vi "Autonomous Independent.vi"() -> ()   [LabVIEW 2014]
doc: "This VI is called when autonomous begins, and will automatically be terminated when autonomous ends. You can carry out timed or sensor driven robot movement independently without needing to return to the caller."
uses:
  <vilib>/Rock Robotics/WPI/Joystick/WPI_JoystickGetSetRefNum.vi
  <vilib>/Rock Robotics/Network Tables/SD Write Numeric Array.vi
  <vilib>/Rock Robotics/WPI/RobotDrive/WPI_RobotDriveGetSetRefNum.vi
  <vilib>/Rock Robotics/WPI/RobotDrive/WPI_RobotDriveMecanumDrive_Cartesian.vi
panel:
  out "Right Rear":dbl
  out "Left Rear":dbl
  out "Right Front":dbl
  out "left Front":dbl
  in  "Deceleration Rate":dbl
  in  "Stop Point":dbl
  in  "Default Output":dbl
  out "Y output":dbl(graph)
  out "Y output":dbl
  in  "Reset Encoder":bool
  in  "Reset Gyro":bool
  out "Angle":dbl
  in  "Angle Constant":dbl
  in  "Angular Rate?":bool
  out "left rear":dbl
  out "left front":dbl
  out "right rear":dbl
  out "right front":dbl
  out "Angular Rate":dbl
  out "average":dbl
  out "Left Rear Encoder 3":dbl
  out "Left Front Encoder 3":dbl
  out "Right Rear Encoder 3":dbl
  out "Right Front Encoder 3":dbl
  out "Average 3":dbl
  out "Gyro 3":dbl
  out "Left Rear Encoder 2":dbl
  out "Left Front Encoder 2":dbl
  out "Right Rear Encoder 2":dbl
  out "Right Front Encoder 2":dbl
  out "Average 2":dbl
  out "Gyro 2":dbl
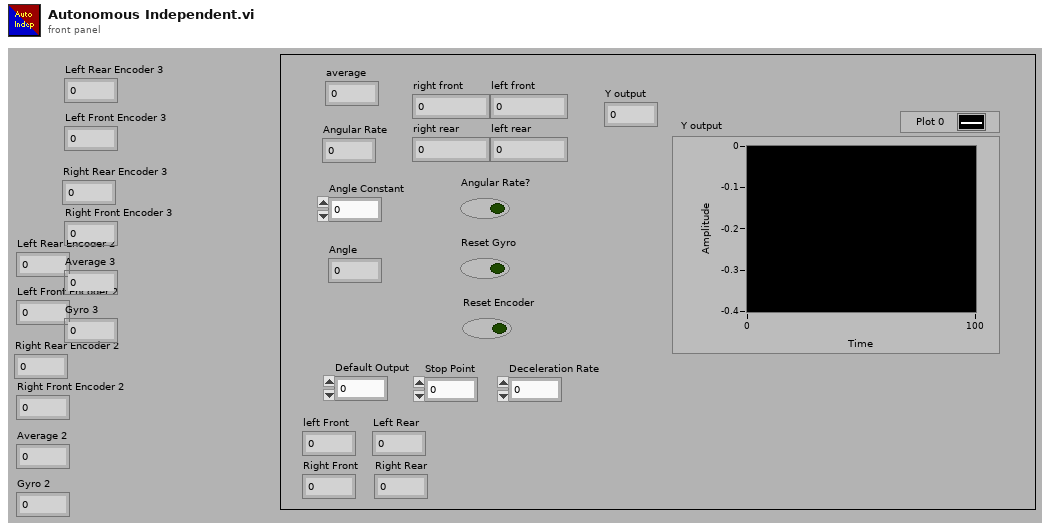
[diagram p1: front panel]
types:
  T1 = typedef "WPI_EncoderDevRef.ctl" = cluster{"DevStatus":errorcluster, "EncoderIndex":T2, "CounterIndex":T3, "DistancePerCount":dbl, "Decoding Type":T4}
  T2 = typedef "FPGA_EncoderIdx.ctl" = enum8{"Enc 0", "Enc 1", "Enc 2", "Enc 3", "Enc 4", "Enc 5", "Enc 6", "Enc 7", "Invalid"}
  T3 = typedef "FPGA_CounterCtrSystemIndex.ctl" = enum8{"Ctr 0", "Ctr 1", "Ctr 2", "Ctr 3", "Ctr 4", "Ctr 5", "Ctr 6", "Ctr 7", "Invalid"}
  T4 = typedef "WPI_EncoderType.ctl" = enum16{"1x", "2x", "4x"}
  T5 = typedef "WPI_GyroDevRef.ctl" = cluster{"DevStatus":errorcluster, "Analog Module":T6, "Analog Channel":T7, "Offset":dbl, "Gain (VoltsPerDegree/Second)":dbl}
  T6 = typedef "FPGA_TypedefAnalogModule.ctl" = enum16{"Controller 1"}
  T7 = typedef "FPGA_AIChannel.ctl" = enum8{"AI 0", "AI 1", "AI 2", "AI 3", "AI MXP 0", "AI MXP 1", "AI MXP 2", "AI MXP 3", "Invalid"}
  T8 = typedef "WPI_RobotDriveDevRef.ctl" = cluster{"DevStatus":errorcluster, "Motors[]":T9[], "Square Inputs":bool, "Max Output":dbl}
  T9 = typedef "WPI_MotorControlDeviceRef.ctl" = cluster{"DeviceStatus":errorcluster, "Type":T10, "PWM":cluster{"Controller":T11, "PWM Channel":T12, "DeadBand":T13}, "CAN":cluster{"Device Number":u8, "Control Mode":T14, "Semaphore":T15, "Max Vout":dbl, "TalonSRX Control Mode":T16}, "Invert":bool, "TransformRef":T17, "InvTransformRef":T17}
  T10 = typedef "WPI_MotorControlType.ctl" = enum16{"PWM", "CAN", "CANTalonSRX"}
  T11 = typedef "FPGA_TypedefDigitalModule.ctl" = enum16{"Controller 1"}
  T12 = typedef "FPGA_DIOPWMChannel.ctl" = enum8{"PWM 0", "PWM 1", "PWM 2", "PWM 3", "PWM 4", "PWM 5", "PWM 6", "PWM 7", "PWM 8", "PWM 9", "PWM MXP 0", "PWM MXP 1", "PWM MXP 2", "PWM MXP 3", "PWM MXP 4", "PWM MXP 5", "PWM MXP 6", "PWM MXP 7", "PWM MXP 8", "PWM MXP 9", "Invalid"}
  T13 = typedef "WPI_PWMDeadband.ctl" = cluster{"Name":string, "maxPositivePwm":i32, "minPositivePwm":i32, "centerPwm":i32, "maxNegativePwm":i32, "minNegativePwm":i32, "angularRange":u16}
  T14 = typedef "WPI_CANJaguar_ControlMode.ctl" = enum8{"Percent VBus", "Current", "Speed", "Position", "Voltage"}
  T15 = typedef "Semaphore RefNum" = refnum<k1>
  T16 = typedef "WPI_CANTalonSRX_APIControlMode.ctl" = enum8{"Percent VBus", "Speed", "Position", "Slave", "Unchanged / Invalid"}
  T17 = typedef "WPI_PWMTransform_ConPane.ctl" = refnum<vi>
  T18 = typedef "WPI_JoystickDevRef.ctl" = cluster{"Device":T19}
  T19 = typedef "WPI_JoystickDeviceEnum.ctl" = enum16{"USB 0", "USB 1", "USB 2", "USB 3", "USB 4", "USB 5"}
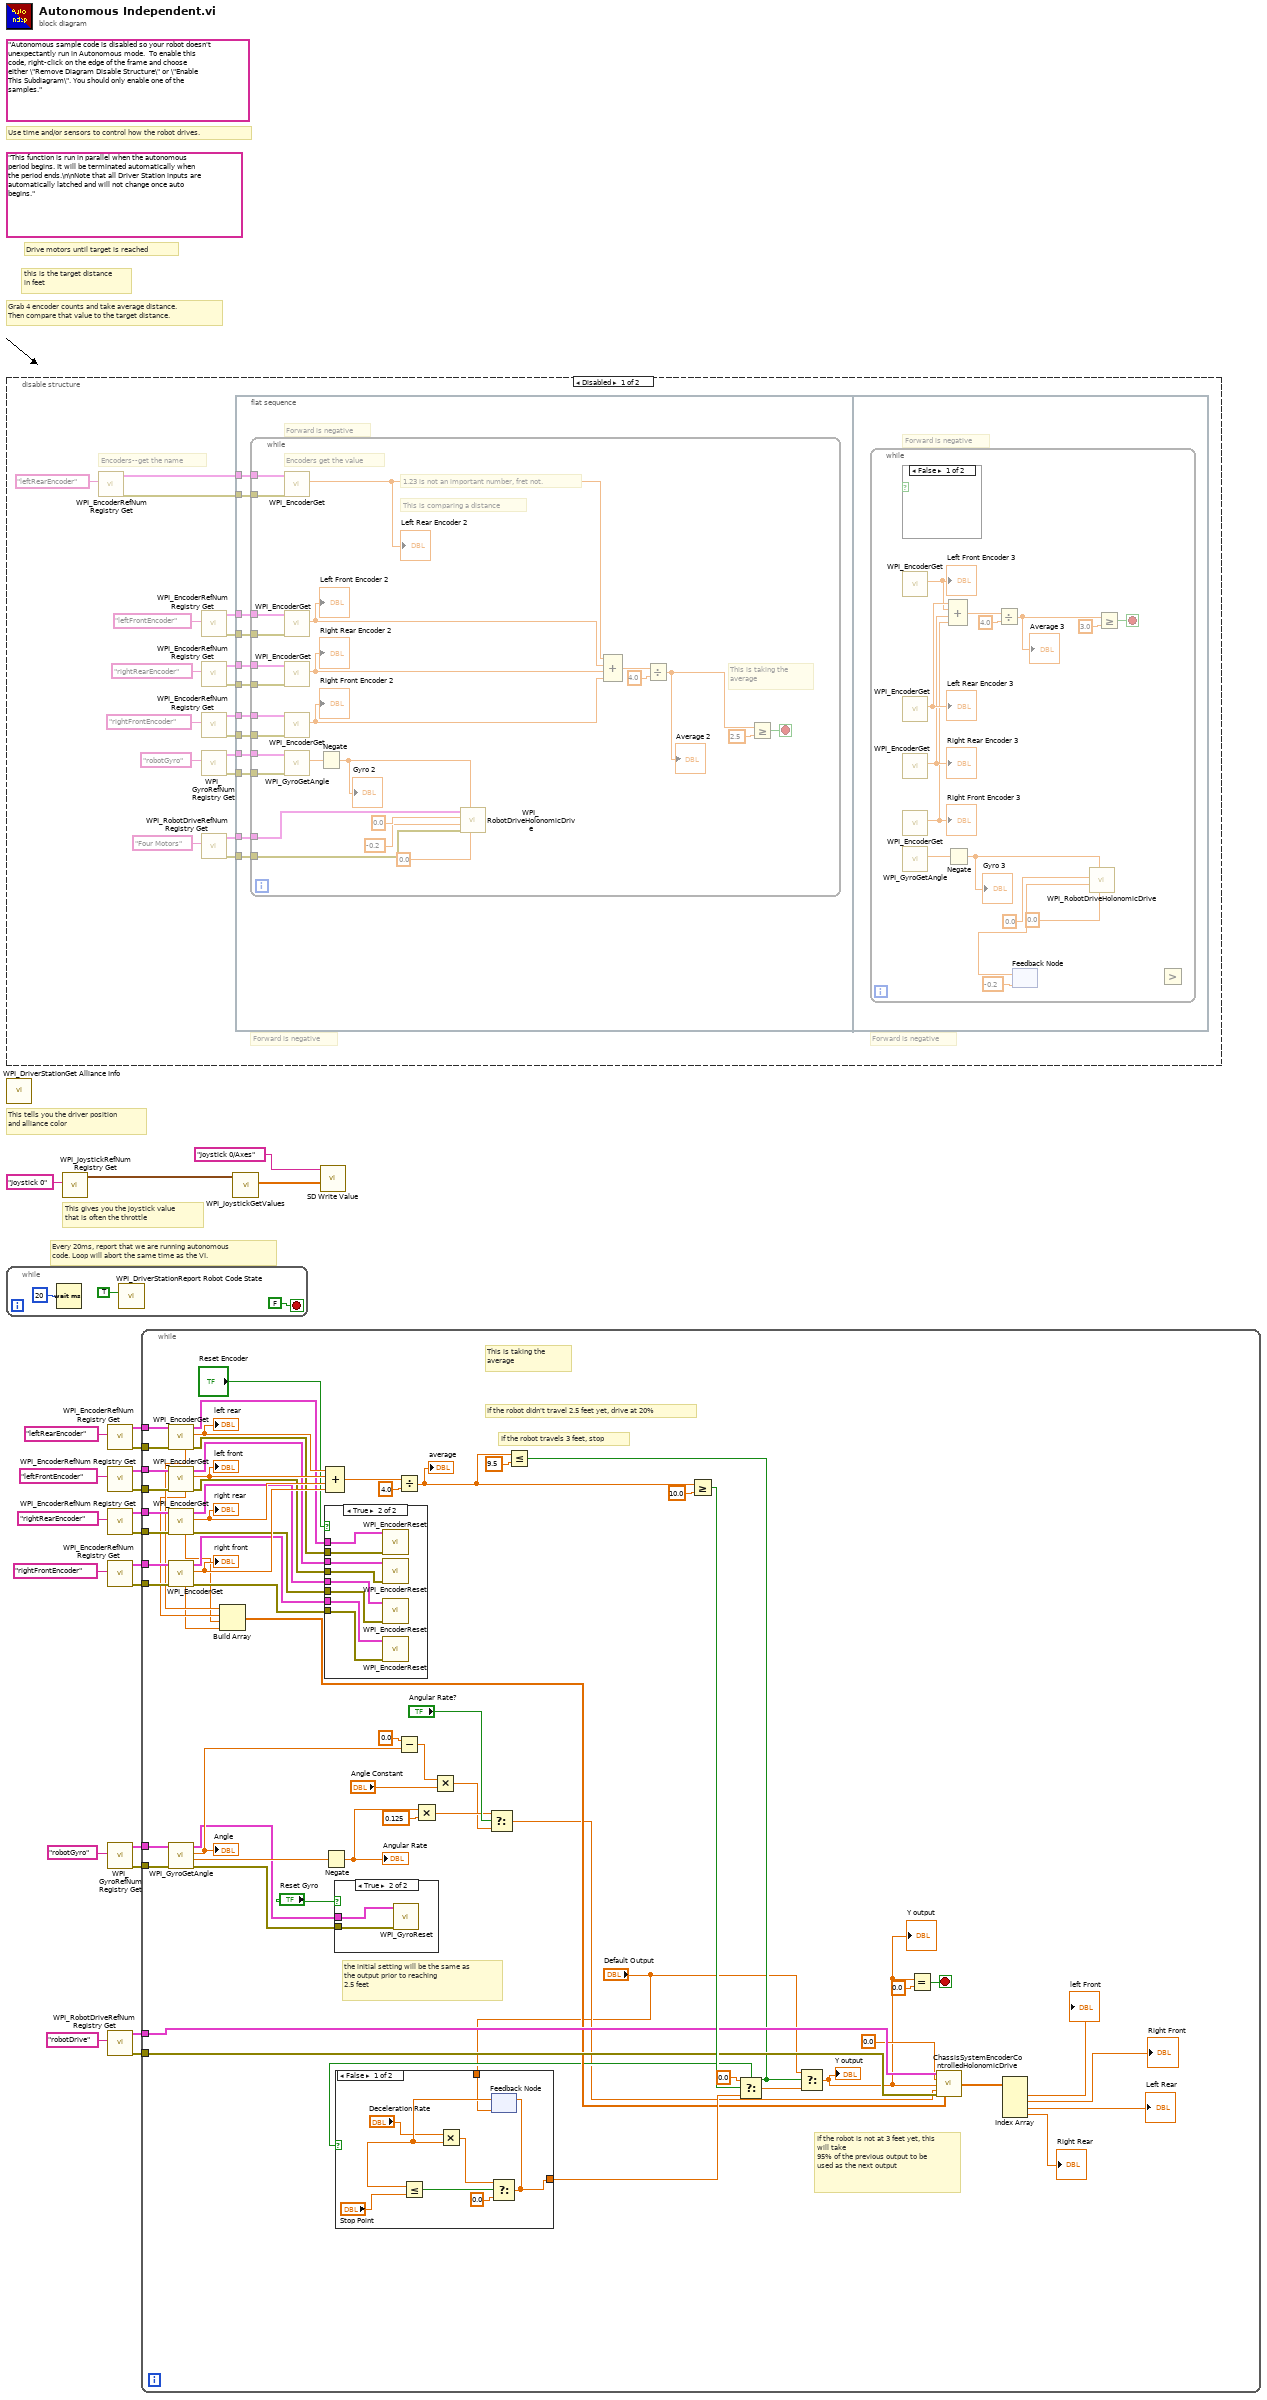
[diagram p0: block diagram]
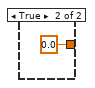
[diagram p2: hidden frame]
diagram:
  (unwired) "Autonomous sample code is disabled so your robot doesn't unexpectantly run in Autonomous mode.  To enable this code, right-click on the edge of the frame and choose either \"Remove Diagram Disable Structure\" or \"Enable This Subdiagram\". You should only enable one of the samples."
  (unwired) "This function is run in parallel when the autonomous period begins. It will be terminated automatically when the period ends.\n\nNote that all Driver Station inputs are automatically latched and will not change once auto begins."
  # "this is the target distance\nin feet"
  # "Drive motors until target is reached"
  # "Grab 4 encoder counts and take average distance.\nThen compare that value to the target distance."
  # "Every 20ms, report that we are running autonomous\ncode. Loop will abort the same time as the VI."
  # "This gives you the joystick value\nthat is often the throttle"
  # "Use time and/or sensors to control how the robot drives."
  # "This tells you the driver position\nand alliance color"
  n1 = disable-structure shown="Disabled" {
    frame Disabled {
      # "Forward is negative"
      # "Forward is negative"
      # "Encoders--get the name"
      n2 = call <vilib>:"WPI_EncoderRefNum Registry Get.vi"("refnum name"="leftRearEncoder") -> ("error out"=w29:errorcluster, "EncoderDevRef"=w30:T1)  [unwired: 9 in]
      n3 = call <vilib>:"WPI_EncoderRefNum Registry Get.vi"("refnum name"="leftFrontEncoder") -> ("error out"=w27:errorcluster, "EncoderDevRef"=w28:T1)  [unwired: 9 in]
      n4 = call <vilib>:"WPI_EncoderRefNum Registry Get.vi"("refnum name"="rightRearEncoder") -> ("error out"=w25:errorcluster, "EncoderDevRef"=w26:T1)  [unwired: 9 in]
      n5 = call <vilib>:"WPI_EncoderRefNum Registry Get.vi"("refnum name"="rightFrontEncoder") -> ("error out"=w24:errorcluster, "EncoderDevRef"=w23:T1)  [unwired: 9 in]
      n6 = call <vilib>:"WPI_GyroRefNum Registry Get.vi"("refnum name"="robotGyro") -> ("error out"=w33:errorcluster, "GyroDevRef"=w34:T5)  [unwired: 9 in]
      n7 = call <vilib>:"WPI_RobotDriveRefNum Registry Get.vi"("refnum name"="Four Motors") -> ("error out"=w31:errorcluster, "RobotDriveDevRef"=w32:T8)  [unwired: 9 in]
      n8 = flat-sequence {
        tunnel: w34 -> [w52]
        tunnel: w33 -> [w51]
        tunnel: w32 -> [w50]
        tunnel: w31 -> [w49]
        tunnel: w30 -> [w48]
        tunnel: w29 -> [w47]
        tunnel: w28 -> [w46]
        tunnel: w27 -> [w45]
        tunnel: w26 -> [w44]
        tunnel: w25 -> [w43]
        tunnel: w24 -> [w42]
        tunnel: w23 -> [w41]
        frame #0 {
          # "Forward is negative"
          n9 = while {
            tunnel: w52 -> [w60]
            tunnel: w51 -> [w59]
            tunnel: w50 -> [w58]
            tunnel: w49 -> [w57]
            tunnel: w48 -> [w71]
            tunnel: w47 -> [w70]
            tunnel: w46 -> [w69]
            tunnel: w45 -> [w68]
            tunnel: w44 -> [w67]
            tunnel: w43 -> [w66]
            tunnel: w41 -> [w65]
            tunnel: w42 -> [w64]
            stop <- w63 stop-if-true
            # "Encoders get the value"
            # "This is comparing a distance"
            # "This is taking the average"
            # "1.23 is not an important number, fret not."
            n10 = call <vilib>:"WPI_EncoderGet.vi"("error in (no error)"=w70, "EncoderDevRef"=w71) -> ("Distance"=w75:dbl)  [unwired: 4 in, 5 out]
            "Left Rear Encoder 2" <- w75
            n11 = call <vilib>:"WPI_EncoderGet.vi"("error in (no error)"=w68, "EncoderDevRef"=w69) -> ("Distance"=w74:dbl)  [unwired: 4 in, 5 out]
            "Left Front Encoder 2" <- w74
            n12 = call <vilib>:"WPI_EncoderGet.vi"("error in (no error)"=w66, "EncoderDevRef"=w67) -> ("Distance"=w73:dbl)  [unwired: 4 in, 5 out]
            "Right Rear Encoder 2" <- w73
            n13 = call <vilib>:"WPI_EncoderGet.vi"("error in (no error)"=w64, "EncoderDevRef"=w65) -> ("Distance"=w72:dbl)  [unwired: 4 in, 5 out]
            "Right Front Encoder 2" <- w72
            n14 = call <vilib>:"WPI_GyroGetAngle.vi"("error in (no error)"=w59, "GyroDevRef"=w60) -> ("Angle"=w56:dbl)  [unwired: 6 in, 3 out]
            n15 = Negate(x=w56) -> (-x=w55:dbl)
            "Gyro 2" <- w55
            n16 = call-poly <vilib>:"WPI_RobotDriveHolonomicDrive.vi"("Rotation"=0.0, "Gyro Angle"=w55, "error in (no error)"=w57, "Y"=-0.2, "X"=0.0, "RobotDriveDevRef"=w58) -> ()  [unwired: 3 in, 3 out]
            n17 = Compound Arithmetic op=ADD(w75, w74, w73, w72) -> (w77:dbl)
            n18 = Divide(x=w77, y=4.0) -> (x/y=w54:dbl)
            "Average 2" <- w54
            n19 = Greater Or Equal?(x=w54, y=2.5) -> (x >= y?=w63:bool)
          }
        }
        frame #1 {
          # "Forward is negative"
          n20 = while {
            stop <- w86 stop-if-true
            n21 = case shown="False" {
              selector: _ -> [_ _]
              frame False {
              }
              frame True {
              }
            }
            n22 = call <vilib>:"WPI_EncoderGet.vi"() -> ("Distance"=w89:dbl)  [unwired: 6 in, 5 out]
            "Left Front Encoder 3" <- w89
            n23 = call <vilib>:"WPI_EncoderGet.vi"() -> ("Distance"=w90:dbl)  [unwired: 6 in, 5 out]
            "Left Rear Encoder 3" <- w90
            n24 = call <vilib>:"WPI_EncoderGet.vi"() -> ("Distance"=w88:dbl)  [unwired: 6 in, 5 out]
            "Right Rear Encoder 3" <- w88
            n25 = call <vilib>:"WPI_EncoderGet.vi"() -> ("Distance"=w87:dbl)  [unwired: 6 in, 5 out]
            "Right Front Encoder 3" <- w87
            n26 = call <vilib>:"WPI_GyroGetAngle.vi"() -> ("Angle"=w83:dbl)  [unwired: 8 in, 3 out]
            n27 = Negate(x=w83) -> (-x=w82:dbl)
            "Gyro 3" <- w82
            n28 = Compound Arithmetic op=ADD(w90, w89, w88, w87) -> (w92:dbl)
            n29 = Divide(x=w92, y=4.0) -> (x/y=w81:dbl)
            "Average 3" <- w81
            n30 = feedback-in #1() -> ()  [unwired: 1 out]
            n31 = feedback #1(-0.2) -> (w79:dbl)
            n32 = call-poly <vilib>:"WPI_RobotDriveHolonomicDrive.vi"("Rotation"=0.0, "Gyro Angle"=w82, "Y"=w79, "X"=0.0) -> ()  [unwired: 5 in, 3 out]
            n33 = Greater Or Equal?(x=w81, y=3.0) -> (x >= y?=w86:bool)
            n34 = Greater?() -> ()  [unwired: 2 in, 1 out]
          }
        }
      }
    }
    frame Enabled {
    }
  }
  n35 = call <vilib>:"WPI_DriverStationGet Alliance Info.vi"() -> ()  [unwired: 12 out]
  n36 = while {
    stop <- FALSE stop-if-true
    n37 = Wait (ms)(milliseconds to wait=u32 20) -> ()  [unwired: 1 out]
    n38 = call <vilib>:"WPI_DriverStationReport Robot Code State.vi"("Autonomous"=TRUE) -> ()  [unwired: 10 in, 1 out]
  }
  n39 = call <vilib>:"WPI_JoystickRefNum Registry Get.vi"("refnum name"="Joystick 0") -> ("JoystickDevRef"=w21:T18)  [unwired: 1 in, 9 out]
  n40 = call <vilib>:"WPI_EncoderRefNum Registry Get.vi"("refnum name"="leftRearEncoder") -> ("error out"=w14:errorcluster, "EncoderDevRef"=w15:T1)  [unwired: 9 in]
  n41 = call <vilib>:"WPI_EncoderRefNum Registry Get.vi"("refnum name"="leftFrontEncoder") -> ("error out"=w12:errorcluster, "EncoderDevRef"=w13:T1)  [unwired: 9 in]
  n42 = call <vilib>:"WPI_EncoderRefNum Registry Get.vi"("refnum name"="rightRearEncoder") -> ("error out"=w10:errorcluster, "EncoderDevRef"=w11:T1)  [unwired: 9 in]
  n43 = call <vilib>:"WPI_EncoderRefNum Registry Get.vi"("refnum name"="rightFrontEncoder") -> ("error out"=w8:errorcluster, "EncoderDevRef"=w9:T1)  [unwired: 9 in]
  n44 = call <vilib>:"WPI_GyroRefNum Registry Get.vi"("refnum name"="robotGyro") -> ("error out"=w1:errorcluster, "GyroDevRef"=w2:T5)  [unwired: 9 in]
  n45 = call <vilib>:"WPI_RobotDriveRefNum Registry Get.vi"("refnum name"="robotDrive") -> ("error out"=w6:errorcluster, "RobotDriveDevRef"=w7:T8)  [unwired: 9 in]
  n46 = while {
    tunnel: w15 -> [w119]
    tunnel: w14 -> [w155]
    tunnel: w13 -> [w154]
    tunnel: w12 -> [w153]
    tunnel: w11 -> [w152]
    tunnel: w10 -> [w151]
    tunnel: w9 -> [w150]
    tunnel: w8 -> [w149]
    tunnel: w7 -> [w141]
    tunnel: w6 -> [w140]
    tunnel: w2 -> [w136]
    tunnel: w1 -> [w135]
    stop <- w137 stop-if-true
    # "If the robot is not at 3 feet yet, this will take\n95% of the previous output to be used as the next output"
    # "the initial setting will be the same as the output prior to reaching\n2.5 feet"
    # "If the robot travels 3 feet, stop"
    # "If the robot didn't travel 2.5 feet yet, drive at 20%"
    # "This is taking the average"
    n47 = call <vilib>:"WPI_EncoderGet.vi"("error in (no error)"=w155, "EncoderDevRef"=w119) -> ("error out"=w117:errorcluster, "Distance"=w158:dbl, "EncoderDevRef"=w118:T1, "Rate"=w110:dbl)  [unwired: 4 in, 2 out]
    "left rear" <- w158
    n48 = call <vilib>:"WPI_EncoderGet.vi"("error in (no error)"=w153, "EncoderDevRef"=w154) -> ("error out"=w115:errorcluster, "Distance"=w157:dbl, "EncoderDevRef"=w116:T1, "Rate"=w109:dbl)  [unwired: 4 in, 2 out]
    "left front" <- w157
    n49 = call <vilib>:"WPI_EncoderGet.vi"("error in (no error)"=w151, "EncoderDevRef"=w152) -> ("error out"=w113:errorcluster, "Distance"=w156:dbl, "EncoderDevRef"=w114:T1, "Rate"=w108:dbl)  [unwired: 4 in, 2 out]
    "right rear" <- w156
    n50 = call <vilib>:"WPI_EncoderGet.vi"("error in (no error)"=w149, "EncoderDevRef"=w150) -> ("error out"=w111:errorcluster, "Distance"=w148:dbl, "EncoderDevRef"=w112:T1, "Rate"=w107:dbl)  [unwired: 4 in, 2 out]
    "right front" <- w148
    n51 = call <vilib>:"WPI_GyroGetAngle.vi"("error in (no error)"=w135, "GyroDevRef"=w136) -> ("error out"=w121:errorcluster, "Angular Rate"=w134:dbl, "Angle"=w124:dbl, "GyroDevRef"=w122:T5)  [unwired: 6 in]
    "Angle" <- w124
    n52 = Build Array(w110, w109, w108, w107) -> (w106:dbl[])
    n53 = Negate(x=w134) -> (-x=w132:dbl)
    "Angular Rate" <- w132
    n54 = case shown="True" "Reset Encoder" {
      tunnel: w118 -> [_ w177]
      tunnel: w117 -> [_ w176]
      tunnel: w116 -> [_ w175]
      tunnel: w115 -> [_ w174]
      tunnel: w114 -> [_ w173]
      tunnel: w113 -> [_ w172]
      tunnel: w112 -> [_ w171]
      tunnel: w111 -> [_ w170]
      frame False {
      }
      frame True {
        n55 = call <vilib>:"WPI_EncoderReset.vi"("error in (no error)"=w176, "EncoderDevRef"=w177) -> ()  [unwired: 8 in, 2 out]
        n56 = call <vilib>:"WPI_EncoderReset.vi"("error in (no error)"=w174, "EncoderDevRef"=w175) -> ()  [unwired: 8 in, 2 out]
        n57 = call <vilib>:"WPI_EncoderReset.vi"("error in (no error)"=w172, "EncoderDevRef"=w173) -> ()  [unwired: 8 in, 2 out]
        n58 = call <vilib>:"WPI_EncoderReset.vi"("error in (no error)"=w170, "EncoderDevRef"=w171) -> ()  [unwired: 8 in, 2 out]
      }
    }
    n59 = Compound Arithmetic op=ADD(w158, w157, w156, w148) -> (w159:dbl)
    n60 = case shown="True" "Reset Gyro" {
      tunnel: w122 -> [_ w179]
      tunnel: w121 -> [_ w178]
      frame False {
      }
      frame True {
        n61 = call <vilib>:"WPI_GyroReset.vi"("error in (no error)"=w178, "GyroDevRef"=w179) -> ()  [unwired: 8 in, 2 out]
      }
    }
    n62 = Divide(x=w159, y=4.0) -> (x/y=w131:dbl)
    "average" <- w131
    n63 = Subtract(x=0.0, y=w124) -> (x-y=w127:dbl)
    n64 = Multiply(x=w132, y=0.125) -> (x*y=w129:dbl)
    n65 = Multiply(x=w127, y="Angle Constant") -> (x*y=w125:dbl)
    n66 = Select(t=w129, s="Angular Rate?", f=w125) -> (s? t:f=w104:dbl)
    n67 = Less Or Equal?(x=w131, y=9.5) -> (x <= y?=w105:bool)
    n68 = case shown="False" w105 {
      tunnel: "Default Output" -> [w163 _]
      tunnel: [w164 0.0 ("f")] -> w142
      frame False {
        n69 = feedback #2(w163) -> (w166:dbl)
        n70 = Less Or Equal?(x=w166, y="Stop Point") -> (x <= y?=w168:bool)
        n71 = Multiply(x="Deceleration Rate", y=w166) -> (x*y=w165:dbl)
        n72 = Select(t=w165, s=w168, f=0.0) -> (s? t:f=w164:dbl)
        n73 = feedback-in #2(w164) -> ()
      }
      frame True {
      }
    }
    n74 = Greater Or Equal?(x=w131, y=10.0) -> (x >= y?=w145:bool)
    n75 = Select(t=0.0, s=w145, f=w142) -> (s? t:f=w144:dbl)
    n76 = Select(t="Default Output", s=w105, f=w144) -> (s? t:f=w103:dbl)
    "Y output" <- w103
    "Y output" <- w103
    n77 = Equal?(x=w103, y=0.0) -> (x = y?=w137:bool)
    n78 = call "ChassisSystemEncoderControlledHolonomicDrive.vi"("RobotDriveDevRef"=w141, "X"=0.0, "Y"=w103, "Rotation"=w104, "error in (no error)"=w140, "Encoder Readings"=w106) -> ("Motor Values"=w101:dbl[])  [unwired: 7 in, 2 out]
    n79 = Index Array(array=w101) -> (element #1=→"left Front":dbl, element #2=→"Right Front":dbl, element #3=→"Left Rear":dbl, element #4=→"Right Rear":dbl)  [unwired: 4 in]
  }
  n80 = call <vilib>:"WPI_JoystickGetValues.vi"("JoystickDevRef"=w21) -> ("Axes"=w19:dbl[])  [unwired: 6 in, 4 out]
  n81 = call-poly <vilib>:"SD Write Value.vi"("Numeric Array"=w19, "Name"="Joystick 0/Axes") -> ()  [unwired: 8 in, 2 out]
